vi "VISAResourceName.vi"() -> ()   [LabVIEW 2009]
panel:
  in  "VISA resource name":refnum<visa-resource-name>="USB_Serial"
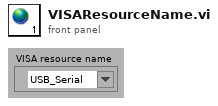
[diagram p1: front panel]
diagram:
